vi "Get Scalar Data Variant.vi"(8 "error in (no error)":errorcluster, 9 "index":i32, 11 "Core Groups Configuration in":refnum<class "Core Groups Configuration.lvclass">) -> (0 "error out":errorcluster, 1 "data version":T1, 2 "data":variant, 3 "Core Groups Configuration out":refnum<class "Core Groups Configuration.lvclass">)   [LabVIEW 2017, in "DSF Core.lvlib" / "Core Groups Configuration.lvclass"]
uses:
  Core Groups Configuration.lvclass
  C:/Git/DSF/Core/Classes/Configuration/Configuration.lvclass
  Typedefs/DSF Version Info.ctl
  Configuration.lvclass
  DSF Core.lvlib
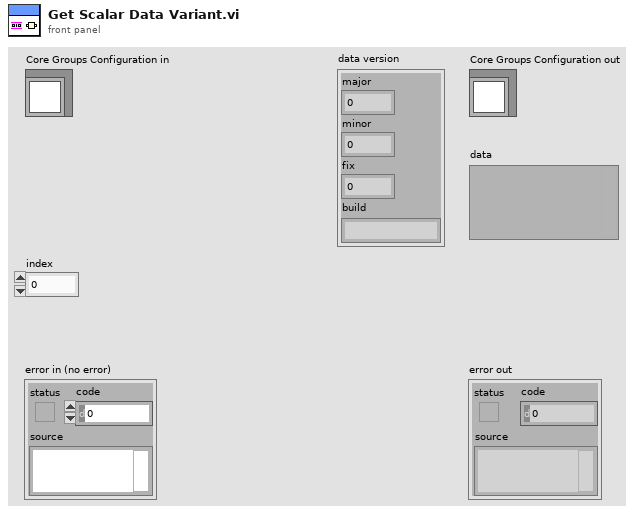
[diagram p1: front panel]
types:
  T1 = typedef "DSF Core.lvlib/DSF Version Info.ctl" = cluster{"major":i32, "minor":i32, "fix":i32, "build":string}
  T2 = typedef "DSF Core.lvlib/Core Groups Configuration.lvclass/Configuration.ctl" = cluster{"name":string, "direction":T3, "cycle timing":T4, "timeout behavior":T5, "convert buffers":bool}
  T3 = typedef "DSF Core.lvlib/DSF Direction.ctl" = enum8{"Tx", "Rx"}
  T4 = typedef "DSF Core.lvlib/DSF Timing Info.ctl" = cluster{"priority":u64, "decimation":u64, "offset":u64}
  T5 = typedef "DSF Core.lvlib/DSF Timeout Behavior.ctl" = enum8{"Increment Late Count", "Throw Error"}
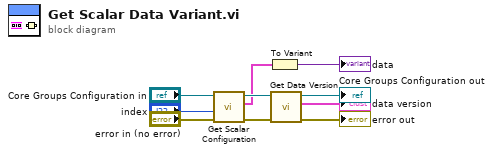
[diagram p0: block diagram]
diagram:
  n1 = call "Get Scalar Configuration.vi"("error in (no error)"="error in (no error)", "index"="index", "Core Groups Configuration in"="Core Groups Configuration in") -> ("error out"=w7:errorcluster, "group configuration"=w2:T2, "Core Groups Configuration out"=w6:refnum<class "Core Groups Configuration.lvclass">)  [unwired: 6 in]
  n2 = To Variant(anything=w2) -> (Variant=→"data":variant)
  n3 = call "Get Data Version.vi"("error in (no error)"=w7, "Configuration in"=w6) -> ("error out"=→"error out":errorcluster, "data version"=→"data version":T1, "Configuration out"=→"Core Groups Configuration out":refnum<class "Core Groups Configuration.lvclass">)  [unwired: 7 in]
